vi "HEWH Check Heating Control Mode.vi"(11 "Flow Event":u16) -> (3 "Large Flag Detected":bool)   [LabVIEW 2016]
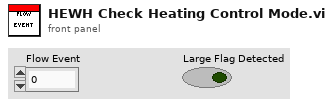
[diagram p1: front panel]
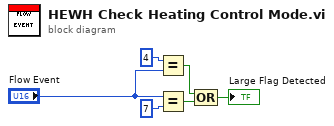
[diagram p0: block diagram]
diagram:
  n1 = Equal?(x=u16 4, y="Flow Event") -> (x = y?=w3:bool)
  n2 = Equal?(x="Flow Event", y=u16 7) -> (x = y?=w2:bool)
  n3 = Compound Arithmetic op=OR(w3, w2) -> (→"Large Flag Detected":bool)
